vi "Energized Picture.vi"(5 "Unused":bool, 10 "Energized State":T2, 11 "Energized Pictures":T3) -> (2 "Energized Picture":T1)   [LabVIEW 2020, in "VolatusGUIElements.lvlib" / "2WayValveH.lvclass"]
uses:
  2WayValveH.lvclass
  Energized Pictures.ctl
  Picture.ctl
  Channel State.ctl
  2WayValveH.lvclass/2WayValveH.ctl
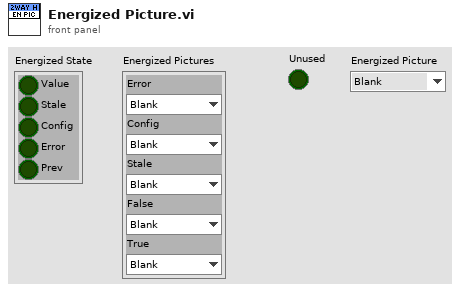
[diagram p1: front panel]
types:
  T1 = typedef "VolatusGUIElements.lvlib/2WayValveH.lvclass/Picture.ctl" = enum16{"Blank", "OutClose", "OutOpen", "OutTranClose", "OutTranOpen", "OutConfig", "OutStale", "OutError", "InClose", "InOpen", "InTranClose", "InTranOpen", "InConfig", "InStale", "InError", "EnOff", "EnOn", "EnConfig", "EnStale", "EnError"}
  T2 = typedef "VolatusGUIElements.lvlib/2WayValveH.lvclass/Channel State.ctl" = cluster{"Value":bool, "Stale":bool, "Config":bool, "Error":bool, "Prev":bool}
  T3 = typedef "VolatusGUIElements.lvlib/2WayValveH.lvclass/Energized Pictures.ctl" = cluster{"Error":T1, "Config":T1, "Stale":T1, "False":T1, "True":T1}
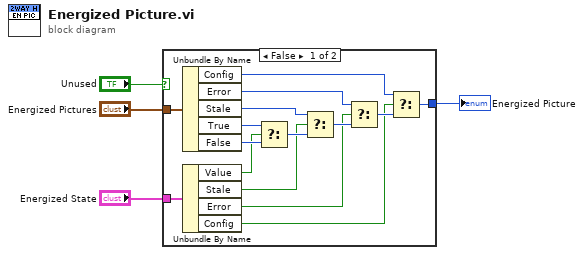
[diagram p0: block diagram]
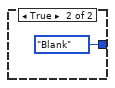
[diagram p2: hidden frame]
diagram:
  n1 = case shown="False" "Unused" {
    tunnel: "Energized Pictures" -> [w19 _]
    tunnel: "Energized State" -> [w18 _]
    tunnel: [w5 Picture."Blank" ("False")] -> w2
    frame False {
      n2 = Unbundle By Name(w19) -> ("Config"=w7:T1, "Error"=w10:T1, "Stale"=w13:T1, "True"=w16:T1, "False"=w17:T1)
      n3 = Unbundle By Name(w18) -> ("Value"=w15:bool, "Stale"=w12:bool, "Error"=w9:bool, "Config"=w6:bool)
      n4 = Select(t=w16, s=w15, f=w17) -> (s? t:f=w14:T1)
      n5 = Select(t=w13, s=w12, f=w14) -> (s? t:f=w11:T1)
      n6 = Select(t=w10, s=w9, f=w11) -> (s? t:f=w8:T1)
      n7 = Select(t=w7, s=w6, f=w8) -> (s? t:f=w5:T1)
    }
    frame True {
    }
  }
  "Energized Picture" <- w2
